vi "Get Veristand Active Version.vi"() -> (3 "Version":string)   [LabVIEW 2019, in "Configuration Tool.lvlib"]
uses:
  Configuration Tool.lvlib
  <vilib>/registry/registry.llb/Registry RtKey.ctl
  <vilib>/registry/registry.llb/Registry SAM.ctl
  <vilib>/registry/registry.llb/Registry View.ctl
  <vilib>/registry/registry.llb/Read Registry Value Simple STR.vi
panel:
  out "Veristand Path":path
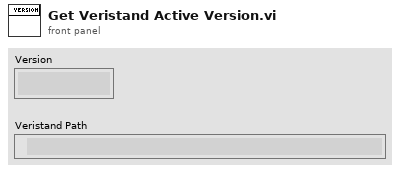
[diagram p1: front panel]
types:
  T1 = typedef "Registry View.ctl" = u16
  T2 = typedef "Registry SAM.ctl" = enum32{"KEY_QUERY_VALUE", "KEY_SET_VALUE", "KEY_CREATE_SUB_KEY", "KEY_ENUMERATE_SUB_KEYS", "KEY_NOTIFY", "KEY_CREATE_LINK", "KEY_READ", "KEY_WRITE", "KEY_ALL_ACCESS", "KEY_READ | KEY_WRITE"}
  T3 = typedef "Registry RtKey.ctl" = enum32{"HKEY_CLASSES_ROOT", "HKEY_CURRENT_USER", "HKEY_LOCAL_MACHINE", "HKEY_USERS", "HKEY_PERFORMANCE_DATA", "HKEY_CURRENT_CONFIG", "HKEY_DYN_DATA"}
  T4 = typedef "Registry refnum.ctl" = refnum<k1>
  T5 = cluster{"numSubKeys":i32, "maxSubKeyLen":i32, "maxSubKeyClassLen":i32}
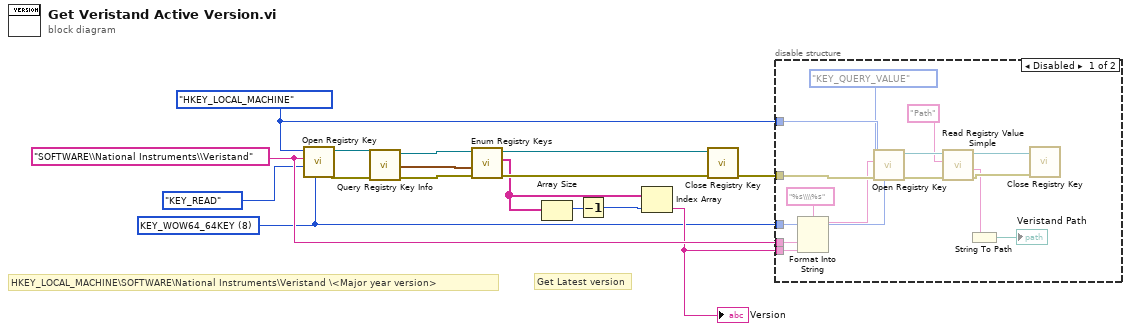
[diagram p0: block diagram]
diagram:
  w4 = T1 8 items=["Default"=0, "KEY_WOW64_64KEY"=8, "KEY_WOW64_32KEY"=9] ("registry view")
  w9 = "SOFTWARE\\National Instruments\\Veristand" ("subkey")
  w6 = Registry_RtKey."HKEY_LOCAL_MACHINE" ("root key (HKEY_LOCAL_MACHINE)")
  # "Get Latest version"
  # "HKEY_LOCAL_MACHINE\\SOFTWARE\\National Instruments\\Veristand \\<Major year version>"
  n1 = call <vilib>:"Open Registry Key.vi"("registry view"=w4, "security access mask (KEY_READ | KEY_WRITE)"=Registry_SAM."KEY_READ", "subkey"=w9, "root key (HKEY_LOCAL_MACHINE)"=w6) -> ("error out"=w15:errorcluster, "refnum out"=w16:T4)  [unwired: 6 in]
  n2 = call <vilib>:"Query Registry Key Info.vi"("error in (no error)"=w15, "refnum"=w16) -> ("error out"=w13:errorcluster, "refnum out"=w14:T4, "subkey info"=w10:T5)  [unwired: 5 in, 2 out]
  n3 = call <vilib>:"Enum Registry Keys.vi"("error in (no error)"=w13, "subkey info"=w10, "refnum"=w14) -> ("error out"=w11:errorcluster, "subkeys"=w3:string[], "refnum out"=w12:T4)  [unwired: 6 in]
  n4 = Array Size(array=w3) -> (size(s)=w2:i32)
  n5 = Decrement(x=w2) -> (x-1=w1:i32)
  n6 = Index Array(array=w3, index=w1) -> (element=w8:string)
  "Version" <- w8
  n7 = call <vilib>:"Close Registry Key.vi"("error in (no error)"=w11, "refnum"=w12) -> ("error out"=w7:errorcluster)  [unwired: 5 in]
  n8 = disable-structure shown="Disabled" {
    disable-tunnel: w9 -> [w31 _]
    disable-tunnel: w8 -> [w30 _]
    disable-tunnel: w7 -> [w28 _]
    disable-tunnel: w6 -> [w27 _]
    disable-tunnel: w4 -> [w20 _]
    frame Disabled {
      n9 = Format Into String(format string="%s\\\\%s", w31, w30) -> (resulting string=w26:string)  [unwired: 2 in, 1 out]
      n10 = call <vilib>:"Open Registry Key.vi"("registry view"=w20, "error in (no error)"=w28, "security access mask (KEY_READ | KEY_WRITE)"=Registry_SAM."KEY_QUERY_VALUE", "subkey"=w26, "root key (HKEY_LOCAL_MACHINE)"=w27) -> ("error out"=w24:errorcluster, "refnum out"=w25:T4)  [unwired: 5 in]
      n11 = call-poly <vilib>:"Read Registry Value Simple.vi"("error in (no error)"=w24, "value"="Path", "refnum"=w25) -> ("error out"=w22:errorcluster, "String/Binary data"=w19:string, "refnum out"=w23:T4)  [unwired: 3 in, 1 out]
      n12 = String To Path(string=w19) -> (path=→"Veristand Path":path)
      n13 = call <vilib>:"Close Registry Key.vi"("error in (no error)"=w22, "refnum"=w23) -> ()  [unwired: 5 in, 1 out]
    }
    frame Enabled {
    }
  }
